vi "user_name.vi"() -> ()   [LabVIEW 2024]
panel:
  in  "User Name":string
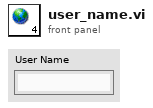
[diagram p1: front panel]
diagram:
